vi "Set.vi"(10 "Bit to set":u8, 11 "Data_In":u16 format="%.0b") -> (3 "Data_Out":u16 format="%.0b")   [LabVIEW 2017, in "Bit Manipulation.lvlib"]
uses:
  Bit Manipulation.lvlib
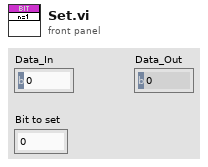
[diagram p1: front panel]
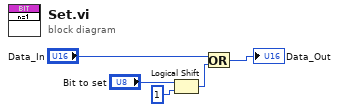
[diagram p0: block diagram]
diagram:
  n1 = Logical Shift(y="Bit to set", x=u16 1) -> (x << y=w3:u16)
  n2 = Or(x="Data_In", y=w3) -> (x .or. y?=→"Data_Out":u16)
